vi "选项名称写入.vi"(8 "error in (no error)":errorcluster caption="错误输入（无错误）", 10 "选项名称":cluster{"索引":i32, "名称":string}, 11 "ScreenSwitching 输入":refnum<class "Screen Switching.lvclass">) -> (0 "error out":errorcluster caption="错误输出", 3 "ScreenSwitching 输出":refnum<class "Screen Switching.lvclass">)   [LabVIEW 2016, in "Screen Switching.lvlib" / "Screen Switching.lvclass"]
uses:
  Screen Switching.lvclass
  Screen Switching.lvclass/Screen Switching.ctl
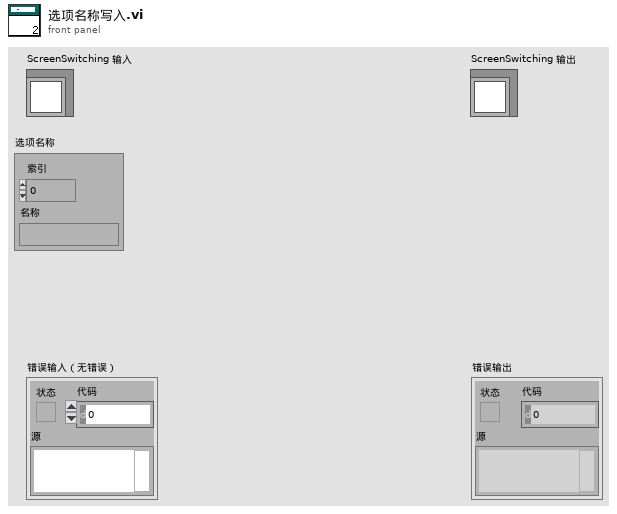
[diagram p1: front panel]
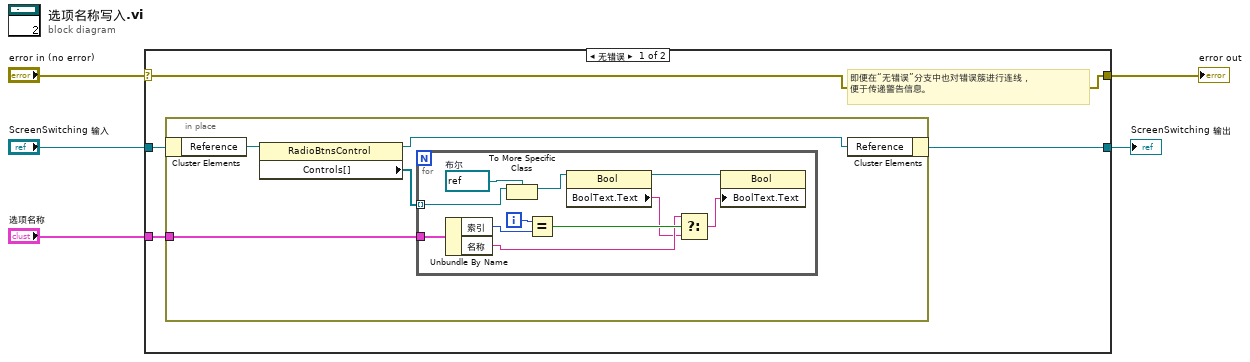
[diagram p0: block diagram]
diagram:
  n1 = case shown="无错误" "error in (no error)" {
    selector: "error in (no error)" -> [w9 w26]
    tunnel: [w9 w26] -> w4
    tunnel: [w7 w25] -> w2
    tunnel: "ScreenSwitching 输入" -> [w8 w25]
    tunnel: "选项名称" -> [w6 _]
    frame No Error {
      # "即便在“无错误”分支中也对错误簇进行连线，\n便于传递警告信息。"
      n2 = in-place {
        in-place-border: w6 -> [w11]
        n3 = in-place-cluster #1(w8) -> ("Reference"=w13:refnum<vi>)
        n4 = property class="RadioBtnsControl"(reference=w13) -> (reference out=w12:refnum<vi>, "Controls[]"=w10:refnum<vi>[])  [unwired: 1 in, 1 out]
        n5 = for {
          tunnel: w10 -> [w24] mode=indexing
          tunnel: w11 -> [w20]
          i -> [w19]
          w23 = refnum<vi> refnum  # 布尔
          n6 = Unbundle By Name(w20) -> ("索引"=w18:i32, "名称"=w16:string)
          n7 = To More Specific Class(target class=w23, reference=w24) -> (specific class reference=w22:refnum<vi>)  [unwired: 1 in, 1 out]
          n8 = Equal?(x=w19, y=w18) -> (x = y?=w17:bool)
          n9 = property class="Bool"(reference=w22) -> (reference out=w21:refnum<vi>, "BoolText.Text"=w15:string)  [unwired: 1 in, 1 out]
          n10 = Select(t=w16, s=w17, f=w15) -> (s? t:f=w14:string)
          n11 = property class="Bool"(reference=w21, "BoolText.Text"=w14) -> ()  [unwired: 1 in, 2 out]
        }
        n12 = in-place-cluster #1("Reference"=w12) -> (w7:refnum<class "Screen Switching.lvclass">)
      }
    }
    frame Error {
    }
  }
  "error out" <- w4
  "ScreenSwitching 输出" <- w2
